vi "Read Value.vi"(8 "error in (no error)":errorcluster, 11 "Boolean Parameter in":refnum<class "File Path Parameter.lvclass">) -> (0 "error out":errorcluster, 2 "Value":path, 3 "Boolean Parameter out":refnum<class "File Path Parameter.lvclass">)   [LabVIEW 2016, in "CD Parameter Manager API.lvlib" / "File Path Parameter.lvclass"]
uses:
  File Path Parameter.lvclass
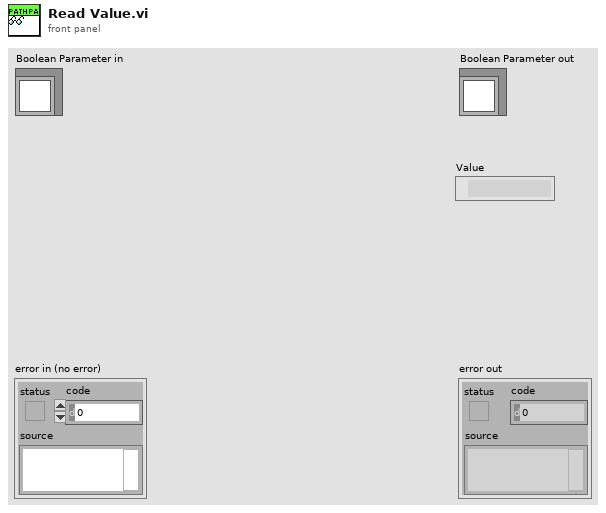
[diagram p1: front panel]
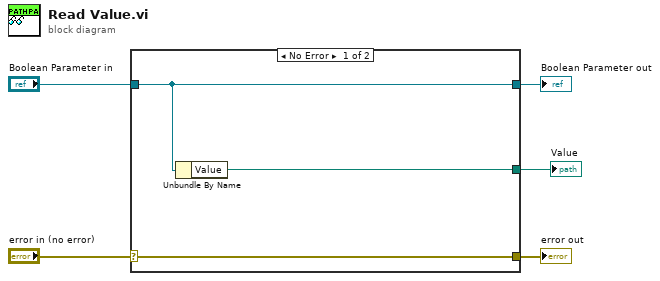
[diagram p0: block diagram]
diagram:
  n1 = case shown="No Error" "error in (no error)" {
    selector: "error in (no error)" -> [w8 w9]
    tunnel: [w8 w9] -> w4
    tunnel: [w7 w10] -> w2
    tunnel: "Boolean Parameter in" -> [w7 w10]
    tunnel: [w6 _] -> w1
    frame No Error {
      n2 = Unbundle By Name(w7) -> ("Value"=w6:path)
    }
    frame Error {
    }
  }
  "error out" <- w4
  "Boolean Parameter out" <- w2
  "Value" <- w1
